vi "多功能采集系统.vi"() -> ()   [LabVIEW 2018]
doc: "该模板用于创建生产者／消费者模式的应用程序。该模板可用于执行诸如数据分析的数据处理，或者在以不均匀速率产生数据的数据源中（如触发采集），当数据可用时对数据进行分析。"
uses:
  <vilib>/Instr/_visa.llb/VISA Configure Serial Port (Instr).vi
panel:
  in  "选项卡控件":enum32{"选项卡 1"}(tab)
  out "跌倒预警灯":bool
  out "温度预警灯":bool
  out "湿度计":dbl(slide) scale=0.0..100.0
  out "温度计":dbl(slide) scale=0.0..100.0
  in  "WebBrowser":refnum<k7>(container) caption="网页浏览器"
  in  "stop":bool caption="停止"
  out "读取缓冲区":string
  in  "地图比例尺":dbl(slide)=15.424242424242424 scale=3.0..18.0
  out "经度":string
  out "纬度":string
  in  "VISA resource name":refnum<visa-resource-name> caption="串口通道"
  out "高度":string
  out "偏航角":string
  out "横滚角":string
  out "俯仰角":string
  out "呼吸声音":string
  out "有毒气体":string
  out "湿度":string
  out "温度":string
  out "成功连接":bool
  out "GPS定位成功":bool
  out "温度图":i32(graph)
  out "毒气图":i32(graph)
  out "声音图":i32(graph)
  out "有毒气体预警灯":bool
  out "呼吸预警灯":bool
  in  "温度阀值":i32
  in  "有毒气体阀值":i32
  in  "呼吸阀值":i32
  out "数组":string[](array[string])
  # "智能消防面罩数据采集系统"
  # "温湿度显示模块"
  # "人体姿态监控模块"
  # "预警灯模块"
  # "有毒气体显示模块"
  # "G\nP\nS\n定位模块"
  # "呼吸监测显示模块"
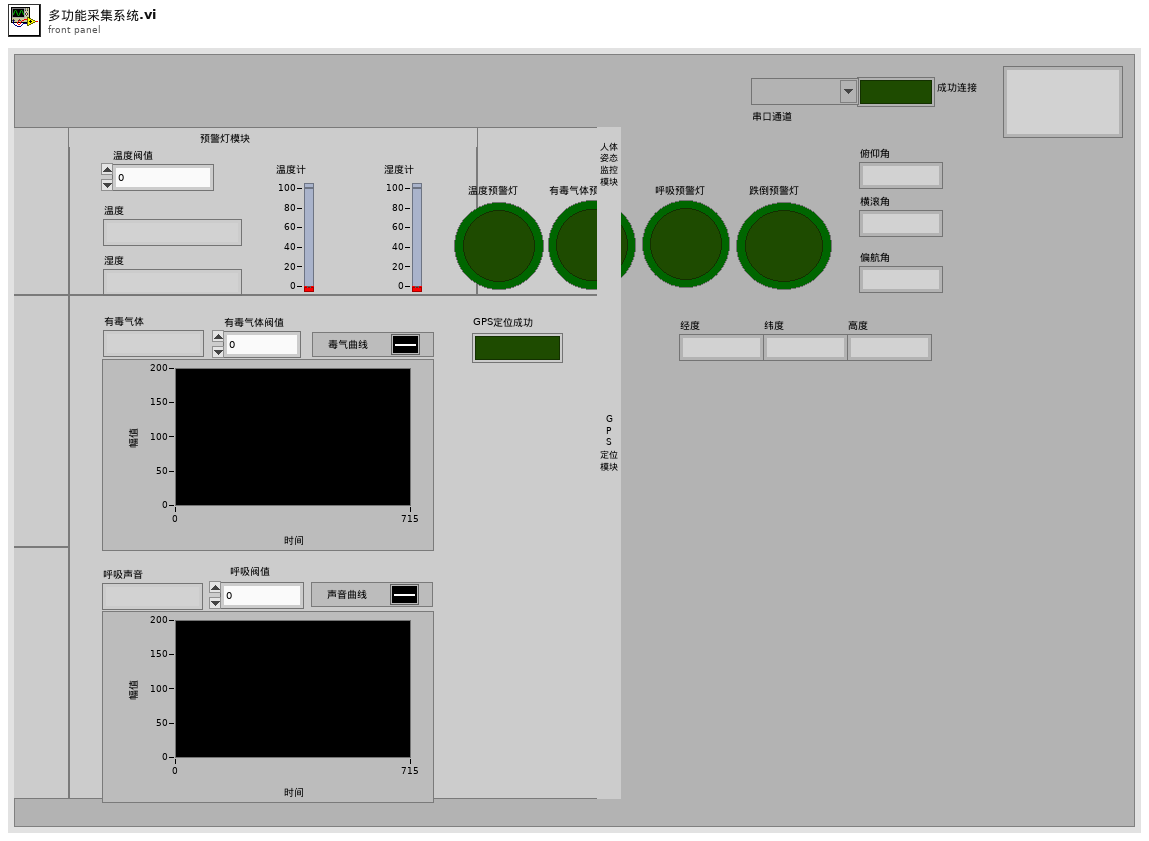
[diagram p1: front panel]
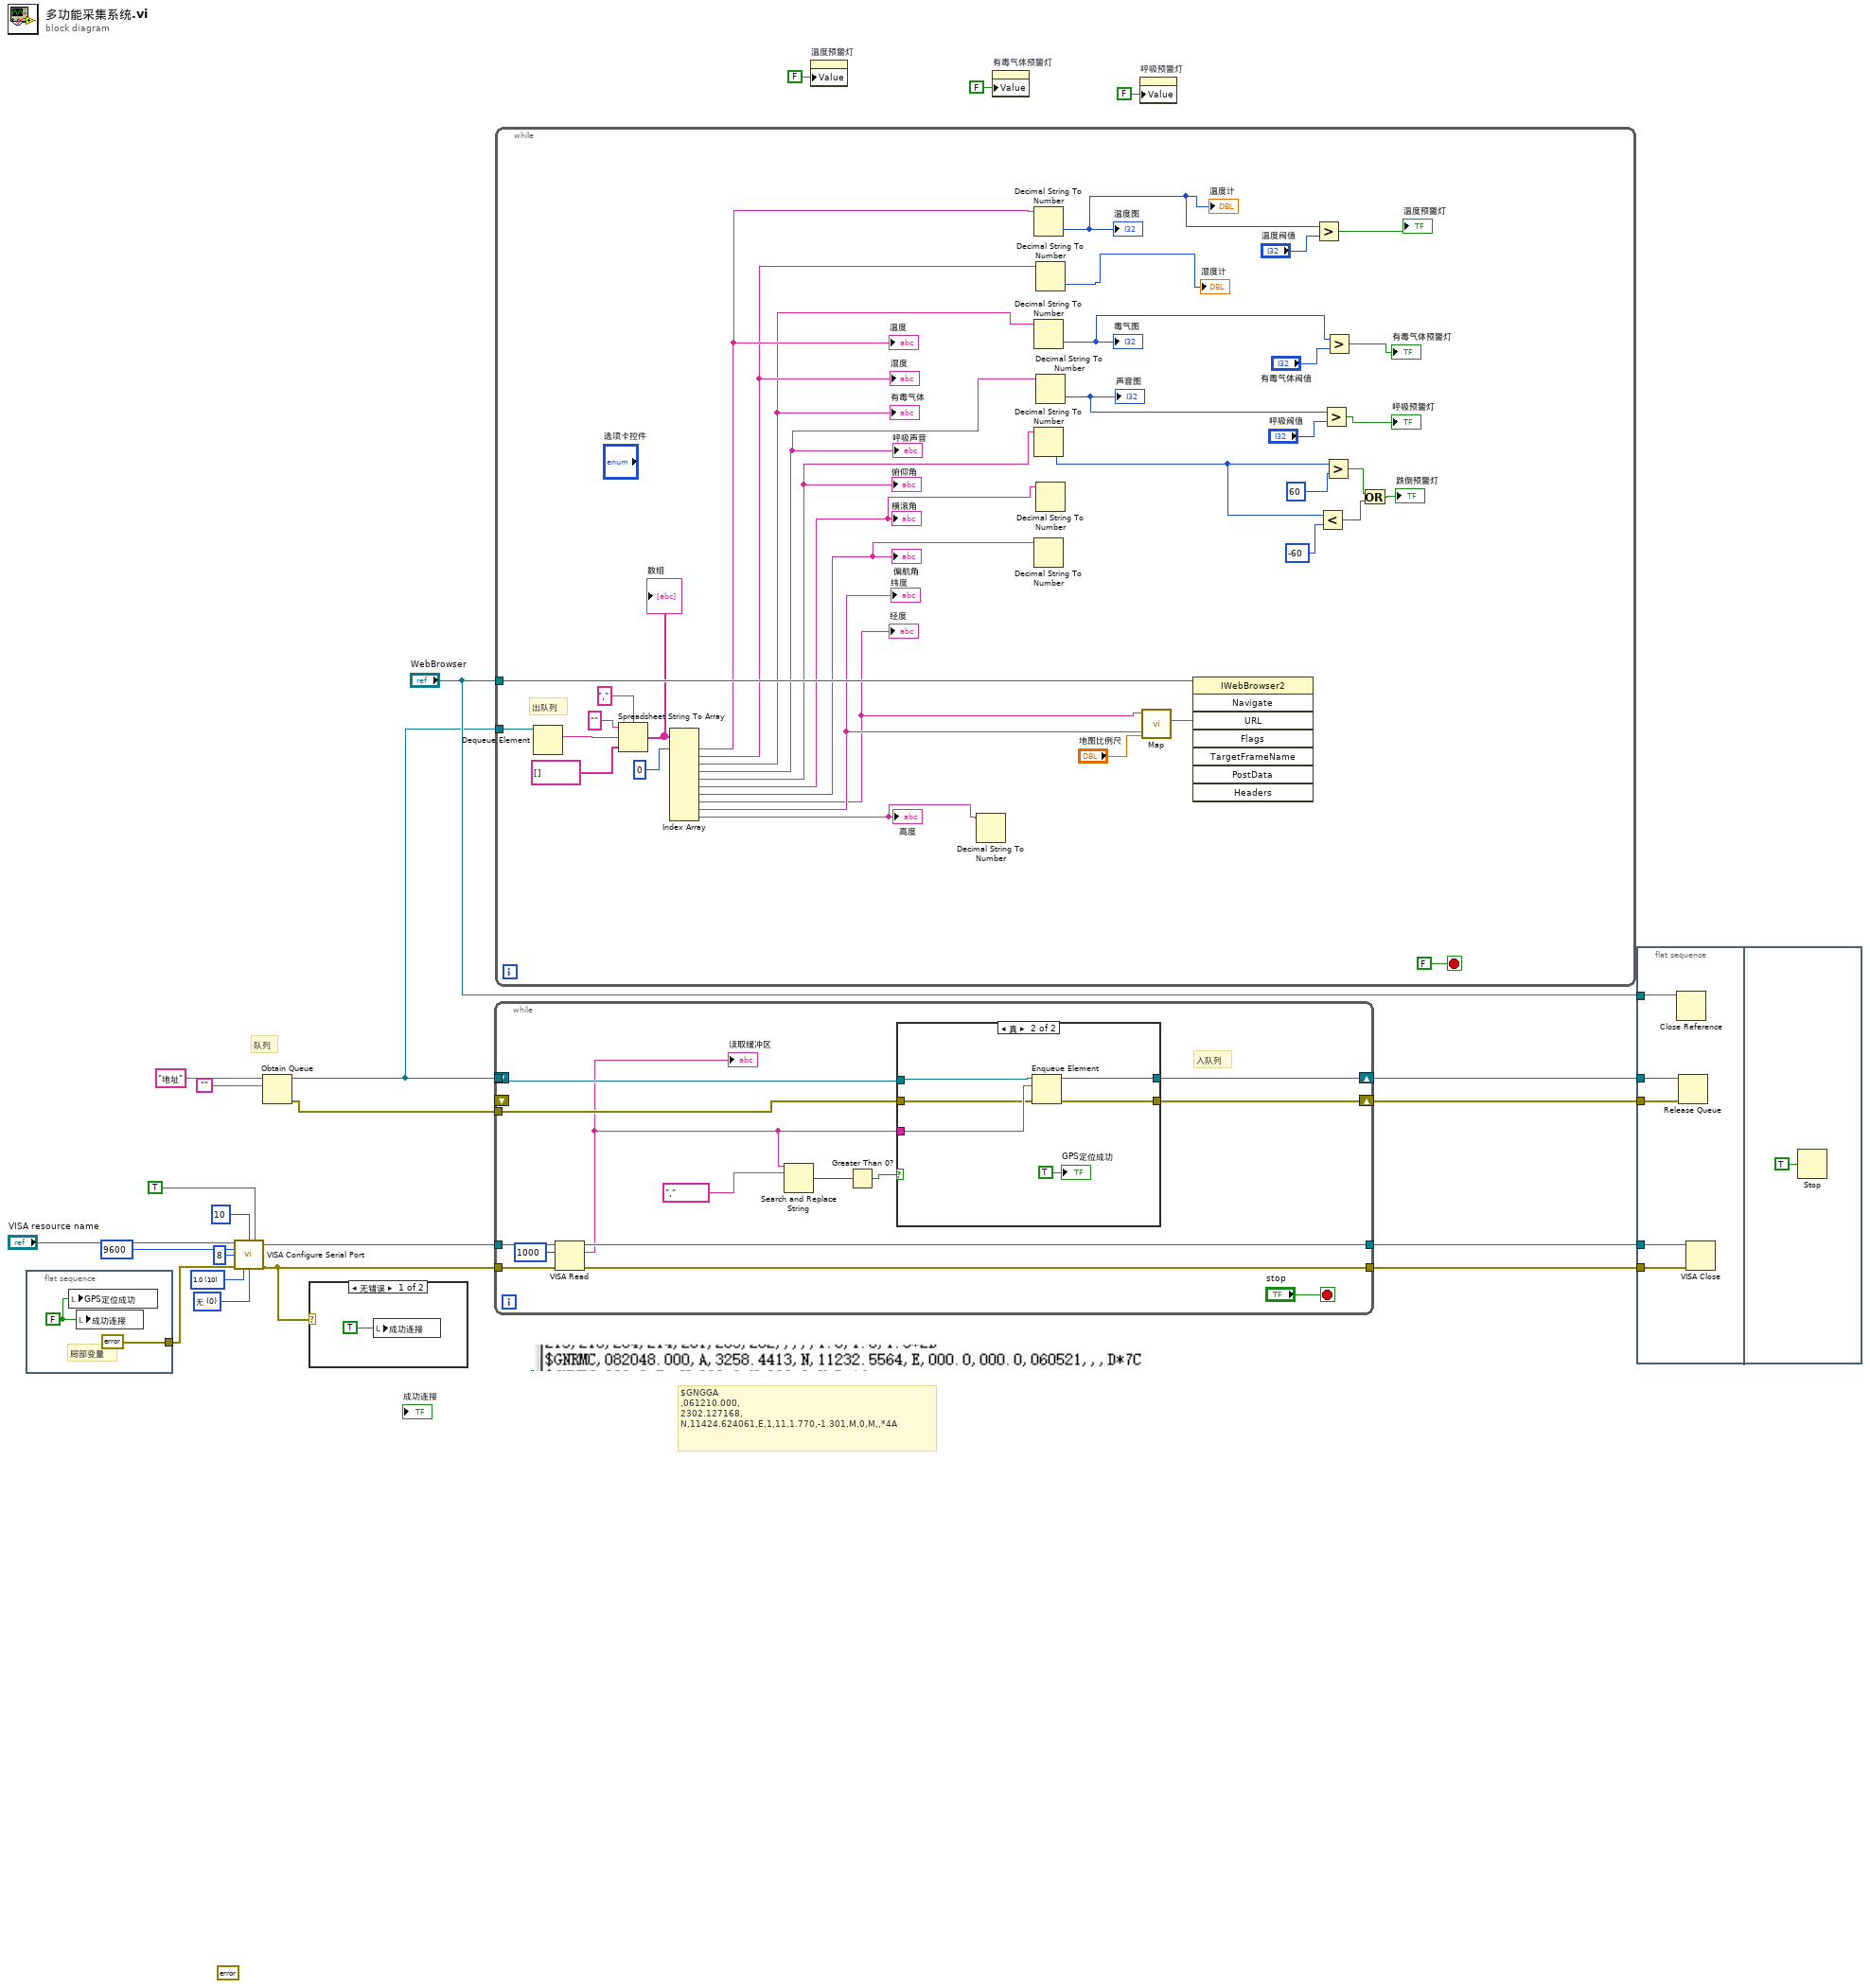
[diagram p0: block diagram]
diagram:
  w6 = u16 0 items=["无", "XON/XOFF", "RTS/CTS", "XON/XOFF & RTS/CTS", "DTR/DSR", "XON/XOFF & DTR/DSR"] ("flow control (0:none)")
  w7 = u16 10 items=["1.0"=10, "1.5"=15, "2.0"=20] ("stop bits (10: 1 bit)")
  (unwired) errorcluster {"status"=FALSE, "code"=0, "source"=""} ("error out")
  # "队列"
  # "$GNGGA\n,061210.000,\n2302.127168,\nN,11424.624061,E,1,11,1.770,-1.301,M,0,M,,*4A"
  n1 = flat-sequence {
    tunnel: [errorcluster {"status"=FALSE, "code"=0, "source"=""} ("错误常量")] -> w13
    frame #0 {
      w23 = FALSE ("4G模块成功")
      # "局部变量"
      n2 = local write "GPS定位成功"(w23) -> ()
      n3 = local write "成功连接"(w23) -> ()
    }
  }
  n4 = call-poly "VISA Configure Serial Port"("VISA resource name"="VISA resource name", "termination char\n(0xA = '\\n' = LF)"=u8 10 ("termination char\n(0xA = '\\n' = LF)"), "Enable Termination\nChar (T)"=TRUE ("Enable Termination\nChar (T)"), "baud rate (9600)"=u32 9600, "data bits (8)"=u16 8, "error in (no error)"=w13, "stop bits (10: 1 bit)"=w7, "flow control (0:none)"=w6) -> ("VISA resource name out"=w15:refnum<visa-resource-name>, "error out"=w14:errorcluster)  [unwired: 6 in]
  n5 = Obtain Queue(name (unnamed)="地址" ("名称（未命名）"), element data type="") -> (queue out=w5:refnum<queue>, error out=w4:errorcluster)  [unwired: 3 in, 1 out]
  n6 = case shown="无错误" w14 {
    frame No Error {
      n7 = local write "成功连接"(TRUE ("4G模块成功")) -> ()
    }
    frame Error {
    }
  }
  n8 = while {
    shift-right: [w30] -> w21
    shift-left: _ -> [_]
    shift-right: [w31] -> w22
    shift-left: _ -> [_]
    tunnel: w15 -> [w38]
    tunnel: w14 -> [w37]
    tunnel: [w35] -> w18
    tunnel: [w36] -> w17
    tunnel: w5 -> [w33]
    tunnel: w4 -> [w32]
    stop <- "stop" stop-if-true
    # "入队列"
    n9 = VISA Read(VISA resource name=w38, byte count=u32 1000 ("字节总数"), error in (no error)=w37) -> (VISA resource name out=w35:refnum<visa-resource-name>, read buffer=w26:string, error out=w36:errorcluster)  [unwired: 1 out]
    "读取缓冲区" <- w26
    n10 = Search and Replace String(input string=w26, search string="," ("搜索字符串/字符(-)")) -> (number of replacements=w29:i32)  [unwired: 6 in, 3 out]
    n11 = Greater Than 0?(x=w29) -> (x > 0?=w27:bool)
    n12 = case shown="真" w27 {
      tunnel: w33 -> [w41 w46]
      tunnel: w26 -> [_ w45]
      tunnel: w32 -> [w40 w44]
      tunnel: [w41 w43] -> w31
      tunnel: [w40 w42] -> w30
      frame False {
      }
      frame True {
        n13 = Enqueue Element(queue=w46, element=w45, error in (no error)=w44) -> (queue out=w43:refnum<queue>, error out=w42:errorcluster)  [unwired: 1 in, 1 out]
        "GPS定位成功" <- TRUE ("GPS定位成功")
      }
    }
  }
  n14 = while {
    tunnel: w5 -> [w84]
    tunnel: "WebBrowser" -> [w83]
    stop <- FALSE stop-if-true
    # "出队列"
    n15 = Dequeue Element(queue=w84) -> (element=w79:string)  [unwired: 2 in, 3 out]
    n16 = Spreadsheet String To Array(delimiter (Tab)="," ("分隔符(Tab)"), format string="" ("格式字符串"), spreadsheet string=w79, array type (2D Dbl)=string[] []) -> (array=w75:string[])
    "数组" <- w75
    n17 = Index Array(array=w75, index #1=0 ("索引")) -> (element #1=w71:string, element #2=w70:string, element #3=w69:string, element #4=w68:string, element #5=w67:string, element #6=w66:string, element #7=w65:string, element #8=w72:string, element #9=w73:string, element #10=w64:string)  [unwired: 9 in]
    "经度" <- w72
    "纬度" <- w73
    "高度" <- w64
    "偏航角" <- w65
    "横滚角" <- w66
    "俯仰角" <- w67
    "呼吸声音" <- w68
    "有毒气体" <- w69
    "湿度" <- w70
    "温度" <- w71
    n18 = Decimal String To Number(string=w64) -> ()  [unwired: 2 in, 2 out]
    n19 = Decimal String To Number(string=w71) -> (number=w62:i32)  [unwired: 2 in, 1 out]
    "温度图" <- w62
    "温度计" <- w62
    n20 = Decimal String To Number(string=w69) -> (number=w56:i32)  [unwired: 2 in, 1 out]
    "毒气图" <- w56
    n21 = Decimal String To Number(string=w67) -> (number=w52:i32)  [unwired: 2 in, 1 out]
    n22 = Decimal String To Number(string=w65) -> ()  [unwired: 2 in, 2 out]
    n23 = Decimal String To Number(string=w70) -> (number=→"湿度计":i32)  [unwired: 2 in, 1 out]
    n24 = Decimal String To Number(string=w68) -> (number=w54:i32)  [unwired: 2 in, 1 out]
    "声音图" <- w54
    n25 = Decimal String To Number(string=w66) -> ()  [unwired: 2 in, 2 out]
    n26 = call "Map.vi"("滑动杆"="地图比例尺", "纬度"=w73, "经度"=w72) -> ("连接的字符串"=w82:string)  [unwired: 8 in]
    n27 = invoke class="IWebBrowser2" method="Navigate"(reference=w83, "URL"=w82) -> ()  [unwired: 6 in, 8 out]
    n28 = Greater?(x=w62, y="温度阀值") -> (0:→"温度预警灯":bool)
    n29 = Less?(x=w52, y=-60) -> (x < y?=w49:bool)
    n30 = Greater?(x=w54, y="呼吸阀值") -> (0:→"呼吸预警灯":bool)
    n31 = Greater?(x=w52, y=60) -> (0:w50:bool)
    n32 = Greater?(x=w56, y="有毒气体阀值") -> (0:→"有毒气体预警灯":bool)
    n33 = Or(x=w50, y=w49) -> (x .or. y?=→"跌倒预警灯":bool)
  }
  n34 = property on="温度预警灯" class="Bool (严格)"("Value"=FALSE ("温度报警灯")) -> ()  [unwired: 2 in, 2 out]
  n35 = property on="有毒气体预警灯" class="Bool (严格)"("Value"=FALSE ("有毒报警灯")) -> ()  [unwired: 2 in, 2 out]
  n36 = property on="呼吸预警灯" class="Bool (严格)"("Value"=FALSE ("声音报警灯")) -> ()  [unwired: 2 in, 2 out]
  n37 = flat-sequence {
    tunnel: w22 -> [w89]
    tunnel: w21 -> [w88]
    tunnel: w18 -> [w87]
    tunnel: w17 -> [w86]
    tunnel: "WebBrowser" -> [w85]
    frame #0 {
      n38 = Close Reference(reference=w85) -> ()  [unwired: 1 in, 1 out]
      n39 = Release Queue(queue=w89, error in (no error)=w88) -> ()  [unwired: 1 in, 3 out]
      n40 = VISA Close(VISA resource name=w87, error in (no error)=w86) -> ()  [unwired: 1 out]
    }
    frame #1 {
      n41 = Stop(stop? (T)=TRUE ("停止？(T)")) -> ()
    }
  }
